vi "Waveform Analisys.vi"() -> ()   [LabVIEW 2013]
uses:
  <vilib>/sound2/lvsound2.llb/Sound Data Format.ctl
  <vilib>/sound2/lvsound2.llb/Sampling Mode.ctl
  <vilib>/Analysis/2dsp.llb/Real FFT.vi
  <vilib>/sound2/lvsound2.llb/Sound Input Read (DBL).vi
  <vilib>/Waveform/DWDTOps.llb/DWDT Analog to Digital.vi
  <vilib>/sound2/lvsound2.llb/Sound Output Write (DBL Single).vi
  <vilib>/Analysis/NI_AALPro.lvlib
  <vilib>/ptbypt/NI_PtbyPt.lvlib
panel:
  in  "Filter":dbl(slide) scale=0.0..0.06
  out "Digital Signal":u32[](graph)
  out "data":u8[][](array[numeric])
  out "Y":digitaldata
  out "Distorted Signal":dbl[](graph)
  in  "Distortion":dbl(slide)=1.0 scale=0.0..100.0
  in  "Gain":dbl(slide)=1.0 scale=0.0..50.0
  in  "stop":bool
  out "Clean Signal":waveform(dbl)[](graph)
  in  "I/O format":T1={"sample rate (S/s)"=22050.0, "number of channels"=2, "bits per sample"=16}
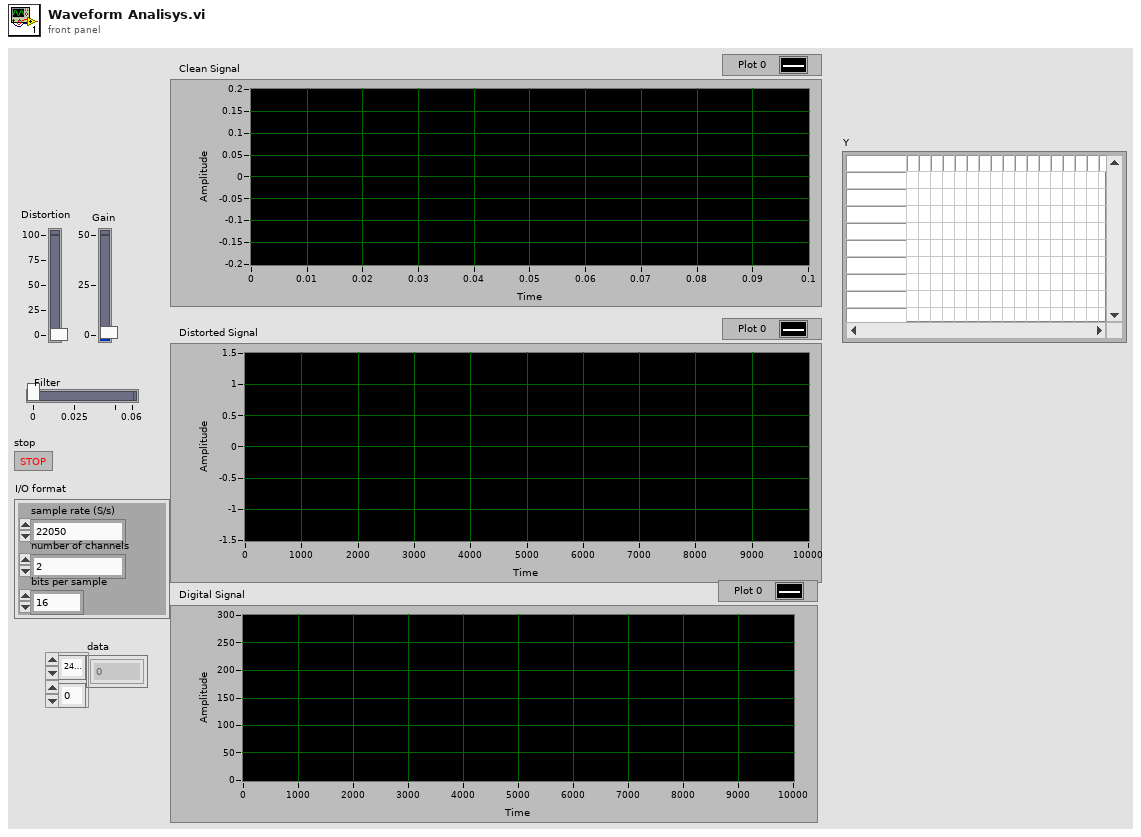
[diagram p1: front panel]
types:
  T1 = typedef "Sound Data Format.ctl" = cluster{"sample rate (S/s)":dbl, "number of channels":i32, "bits per sample":i32}
  T2 = typedef "Sampling Mode.ctl" = i32
  T3 = typedef "Sound Output Task ID.ctl" = u32
  T4 = typedef "Sound Input Task ID.ctl" = u32
  T5 = cluster{"data[0]":waveform(dbl), "data[1]":waveform(dbl), "data[2]":waveform(dbl), "data[3]":waveform(dbl), "data[4]":waveform(dbl), "data[5]":waveform(dbl), "data[6]":waveform(dbl), "data[7]":waveform(dbl), "data[8]":waveform(dbl)}
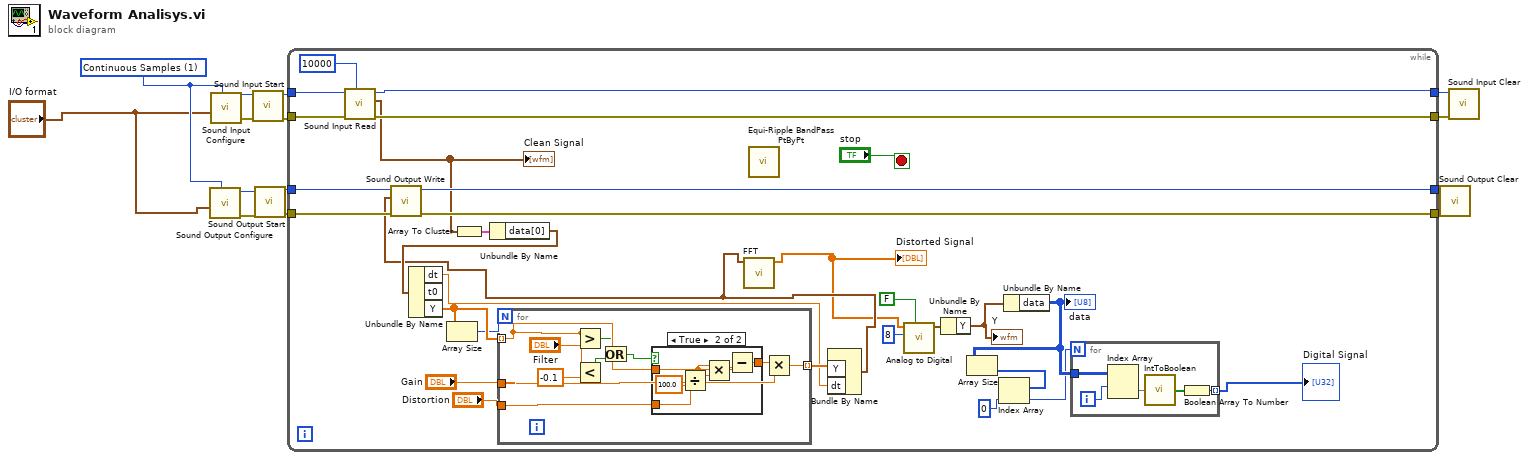
[diagram p0: block diagram]
diagram:
  w2 = T2 1 items=["Finite Samples", "Continuous Samples"] ("sample mode")
  n1 = call <vilib>:"Sound Output Configure.vi"("sample mode"=w2, "sound format"="I/O format") -> ("error out"=w8:errorcluster, "task ID"=w7:T3)  [unwired: 8 in]
  n2 = call <vilib>:"Sound Input Configure.vi"("sample mode"=w2, "sound format"="I/O format") -> ("error out"=w13:errorcluster, "task ID"=w14:T4)  [unwired: 8 in]
  n3 = call <vilib>:"Sound Input Start.vi"("error in (no error)"=w13, "task ID"=w14) -> ("error out"=w11:errorcluster, "task ID out"=w12:T4)  [unwired: 8 in]
  n4 = call <vilib>:"Sound Output Start.vi"("error in (no error)"=w8, "task ID"=w7) -> ("error out"=w5:errorcluster, "task ID out"=w6:T3)  [unwired: 8 in]
  n5 = while {
    tunnel: w12 -> [w44]
    tunnel: w11 -> [w43]
    tunnel: [w42] -> w10
    tunnel: [w41] -> w9
    tunnel: w6 -> [w39]
    tunnel: w5 -> [w38]
    tunnel: [w37] -> w4
    tunnel: [w36] -> w3
    stop <- "stop" stop-if-true
    n6 = call-poly <vilib>:"Sound Input Read.vi"("number of samples/ch"=10000, "error in (no error)"=w43, "task ID"=w44) -> ("error out"=w41:errorcluster, "data"=w35:waveform(dbl)[], "task ID out"=w42:T4)  [unwired: 6 in]
    "Clean Signal" <- w35
    n7 = Array To Cluster(array=w35) -> (cluster=w34:T5)
    n8 = Unbundle By Name(w34) -> ("data[0]"=w28:waveform(dbl))
    n9 = Unbundle By Name(w28) -> ("dt"=w25:dbl, "Y"=w30:dbl[])  [unwired: 1 out]
    n10 = Array Size(array=w30) -> (size(s)=w29:i32)
    n11 = for {
      N: w29 -> [_]
      tunnel: w30 -> [w55] mode=indexing
      tunnel: "Gain" -> [w59]
      tunnel: [w57] -> w32 mode=indexing
      tunnel: "Distortion" -> [w56]
      n12 = Greater?(x=w55, y="Filter") -> (0:w53:bool)
      n13 = Less?(x=w55, y=-0.1) -> (x < y?=w52:bool)
      n14 = Or(x=w53, y=w52) -> (x .or. y?=w51:bool)
      n15 = case shown="True" w51 {
        tunnel: w55 -> [w60 w65]
        tunnel: [w60 w66] -> w58
        tunnel: w56 -> [_ w64]
        frame False {
        }
        frame True {
          n16 = Divide(x=w64, y=100.0) -> (x/y=w61:dbl)
          n17 = Multiply(x=w65, y=w61) -> (x*y=w62:dbl)
          n18 = Subtract(x=w65, y=w62) -> (x-y=w66:dbl)
        }
      }
      n19 = Multiply(x=w58, y=w59) -> (x*y=w57:dbl)
    }
    n20 = call <vilib>:"Equi-Ripple BandPass PtByPt.vi"() -> ()  [unwired: 14 in, 2 out]
    n21 = Bundle By Name("Y"=w32, "dt"=w25) -> (w16:waveform(dbl))  [unwired: 1 in]
    n22 = call-poly <vilib>:"Sound Output Write.vi"("error in (no error)"=w38, "data"=w16, "task ID"=w39) -> ("error out"=w36:errorcluster, "task ID out"=w37:T3)  [unwired: 7 in]
    n23 = call-poly <vilib>:"FFT.vi"("X"=w16) -> ("FFT {X}"=w15:cdb[])  [unwired: 9 in, 1 out]
    "Distorted Signal" <- w15
    n24 = call-poly <vilib>:"Analog to Digital.vi"("compress digital (T)"=FALSE, "resolution (16 bit)"=8, "analog waveform"=w15) -> ("digital waveform"=w24:digitalwaveform)  [unwired: 5 in, 3 out]
    n25 = Unbundle By Name(w24) -> ("Y"=w23:digitaldata)
    "Y" <- w23
    n26 = Unbundle By Name(w23) -> ("data"=w22:u8[][])
    "data" <- w22
    n27 = Array Size(array=w22) -> (size(s)=w21:i32[])
    n28 = Index Array(array=w21, index=0) -> (element=w19:i32)
    n29 = for {
      N: w19 -> [_]
      tunnel: w22 -> [w49]
      tunnel: [w46] -> w18 mode=indexing
      i -> [w45]
      n30 = Index Array(array=w49, index (row)=w45) -> (element=w48:u8[])  [unwired: 1 in]
      n31 = call "IntToBoolean.vi"("Input Int"=w48) -> ("Output Boolean"=w47:bool[])
      n32 = Boolean Array To Number(Boolean array=w47) -> (number=w46:u32)
    }
    "Digital Signal" <- w18
  }
  n33 = call <vilib>:"Sound Output Clear.vi"("error in (no error)"=w3, "task ID"=w4) -> ()  [unwired: 9 in, 1 out]
  n34 = call <vilib>:"Sound Input Clear.vi"("error in (no error)"=w9, "task ID"=w10) -> ()  [unwired: 9 in, 1 out]
